vi "ReAverage Mean.vi"(1 "Lower  Array":dbl[](array[numeric])) -> (0 "mean":dbl format="%0.2f")   [LabVIEW 2009]
uses:
  <vilib>/Analysis/NI_AALBase.lvlib
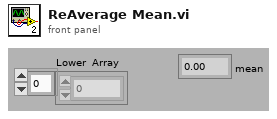
[diagram p1: front panel]
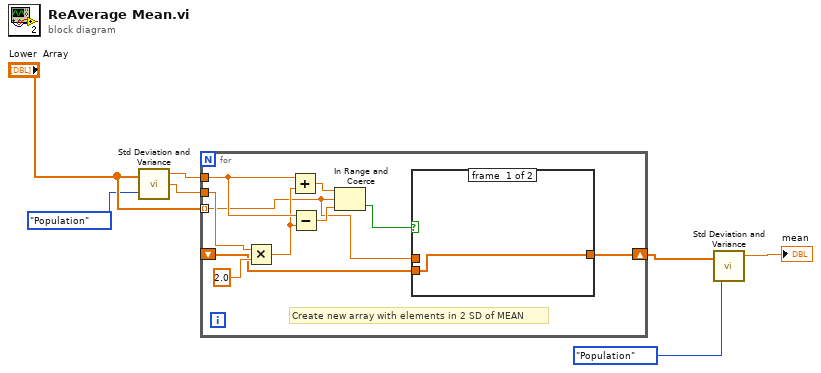
[diagram p0: block diagram]
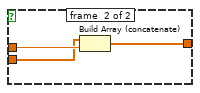
[diagram p2: hidden frame]
diagram:
  n1 = call <vilib>:"Std Deviation and Variance.vi"("X"="Lower  Array", "Weighting (Sample)"=enum16{"Sample", "Population"}."Population") -> ("mean"=w3:dbl, "standard deviation"=w4:dbl)  [unwired: 1 out]
  n2 = for {
    tunnel: "Lower  Array" -> [w10] mode=indexing
    tunnel: w3 -> [w17]
    tunnel: w4 -> [w15]
    shift-right: [w9] -> w5
    shift-left: _ -> [w8]
    # "Create new array with elements in 2 SD of MEAN"
    n3 = Multiply(x=w15, y=2.0) -> (x*y=w14:dbl)
    n4 = Add(x=w17, y=w14) -> (x+y=w13:dbl)
    n5 = Subtract(x=w17, y=w14) -> (x-y=w12:dbl)
    n6 = In Range and Coerce(upper limit=w13, x=w10, lower limit=w12) -> (In Range?=w11:bool)  [unwired: 1 out]
    n7 = case shown="False" w11 {
      tunnel: w10 -> [_ w21]
      tunnel: [w18 w20] -> w9
      tunnel: w8 -> [w18 w19]
      frame #0 {
      }
      frame #1 {
        n8 = Build Array (concatenate)(w19, w21) -> (w20:dbl[])
      }
    }
  }
  n9 = call <vilib>:"Std Deviation and Variance.vi"("X"=w5, "Weighting (Sample)"=enum16{"Sample", "Population"}."Population") -> ("mean"=→"mean":dbl)  [unwired: 2 out]
